vi "relative-file-path-finder-test-vi.vi"() -> (0 "Config File":path, 1 "current VI's path":path, 2 "Current VI's folder":path, 3 "Project Folder":path)   [LabVIEW 2021]
panel:
  in  "Stop Button":bool
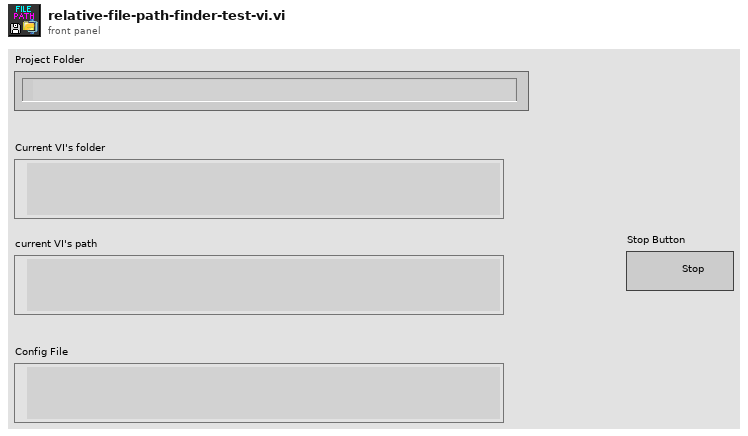
[diagram p1: front panel]
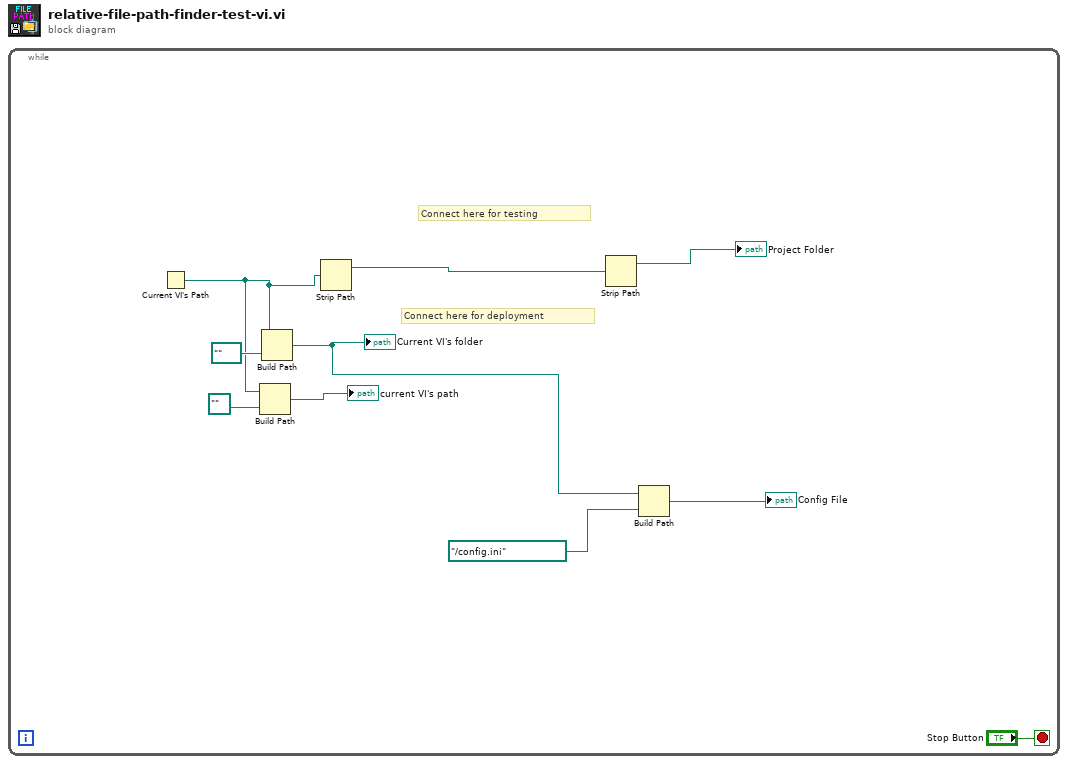
[diagram p0: block diagram]
diagram:
  n1 = while {
    stop <- "Stop Button" stop-if-true
    # "Connect here for deployment"
    # "Connect here for testing"
    n2 = Current VI's Path() -> (path=w5:path)
    n3 = Build Path(base path=w5, name or relative path=path "") -> (appended path=→"current VI's path":path)
    n4 = Build Path(base path=w5, name or relative path=path "..") -> (appended path=w2:path)
    "Current VI's folder" <- w2
    n5 = Strip Path(path=w5) -> (stripped path=w3:path)  [unwired: 1 out]
    n6 = Strip Path(path=w3) -> (stripped path=→"Project Folder":path)  [unwired: 1 out]
    n7 = Build Path(base path=w2, name or relative path=path "../config.ini") -> (appended path=→"Config File":path)
  }
